vi "WriteItemToExcel.vi"(8 "error in (no error)":errorcluster caption="错误输入（无错误）", 9 "Data":string caption="文本", 10 "保存类型":T1, 11 "report in":refnum<class "NI_report.lvclass"> caption="报表输入") -> (0 "error out":errorcluster caption="错误输出", 3 "report out":refnum<class "NI_report.lvclass"> caption="报表输出")   [LabVIEW 2018]
uses:
  ReportItem.ctl
  <vilib>/Utility/NIReport.llb/NI_report.lvclass
  <vilib>/Utility/NIReport.llb/Append Report Text (str wrap).vi
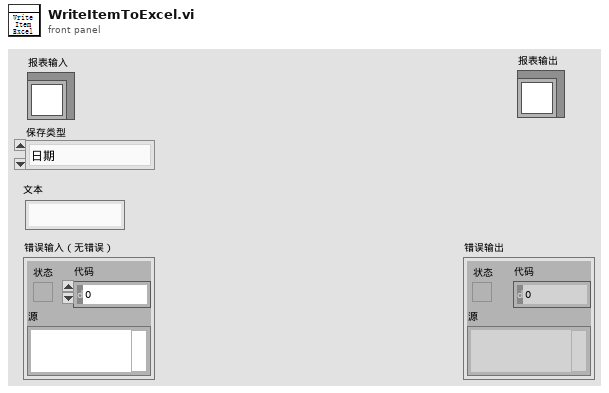
[diagram p1: front panel]
types:
  T1 = typedef "ReportItem.ctl" = enum16{"日期", "激光器编号(Serial)", "功率", "能量", "偏振方向", "偏振度", "脉冲宽度", "脉冲重频", "中心波长", "光谱宽度", "发散角X", "发散角Y", "时间波形路径", "光谱波形路径", "近场图像路径", "远场图像路径", "激光器型号(Type)"}
  T2 = cluster{"position (excel)":cluster{"row":i32, "column":i32}, "name (excel)":string, "bookmark (word)":string}
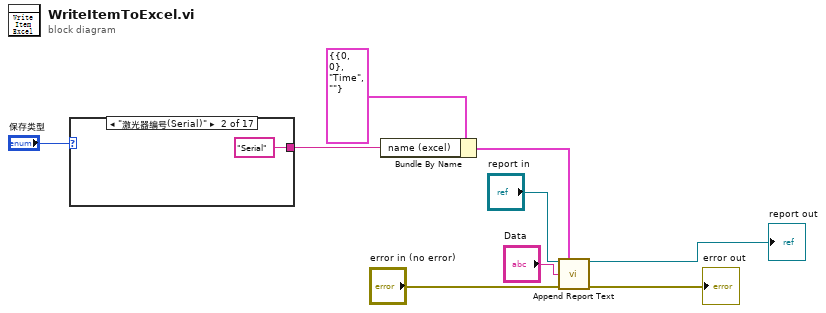
[diagram p0: block diagram]
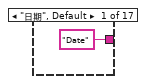
[diagram p2: hidden frame]
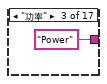
[diagram p3: hidden frame]
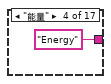
[diagram p4: hidden frame]
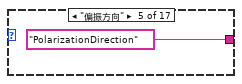
[diagram p5: hidden frame]
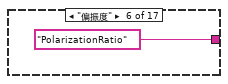
[diagram p6: hidden frame]
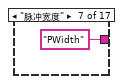
[diagram p7: hidden frame]
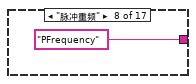
[diagram p8: hidden frame]
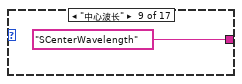
[diagram p9: hidden frame]
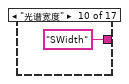
[diagram p10: hidden frame]
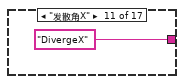
[diagram p11: hidden frame]
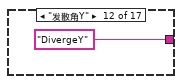
[diagram p12: hidden frame]
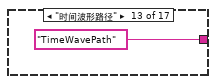
[diagram p13: hidden frame]
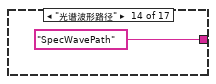
[diagram p14: hidden frame]
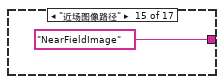
[diagram p15: hidden frame]
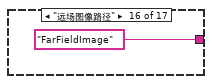
[diagram p16: hidden frame]
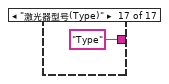
[diagram p17: hidden frame]
diagram:
  n1 = case shown="\"激光器编号(Serial)\"" "保存类型" {
    tunnel: ["Date" "Serial" "Power" "Energy" "PolarizationDirection" "PolarizationRatio" "PWidth" "PFrequency" "SCenterWavelength" "SWidth" "DivergeX" "DivergeY" "TimeWavePath" "SpecWavePath" "NearFieldImage" "FarFieldImage" "Type"] -> w8
    frame "日期", Default {
    }
    frame "激光器编号(Serial)" {
    }
    frame "功率" {
    }
    frame "能量" {
    }
    frame "偏振方向" {
    }
    frame "偏振度" {
    }
    frame "脉冲宽度" {
    }
    frame "脉冲重频" {
    }
    frame "中心波长" {
    }
    frame "光谱宽度" {
    }
    frame "发散角X" {
    }
    frame "发散角Y" {
    }
    frame "时间波形路径" {
    }
    frame "光谱波形路径" {
    }
    frame "近场图像路径" {
    }
    frame "远场图像路径" {
    }
    frame "激光器型号(Type)" {
    }
  }
  n2 = Bundle By Name(cluster=T2 {"position (excel)"={"row"=0, "column"=0}, "name (excel)"="Time", "bookmark (word)"=""} ("MS Office parameters"), "name (excel)"=w8) -> (w7:T2)
  n3 = call-poly <vilib>:"Append Report Text.vi"("report in"="report in", "MS Office parameters"=w7, "text"="Data", "error in (no error)"="error in (no error)") -> ("report out"=→"report out":refnum<class "NI_report.lvclass">, "error out"=→"error out":errorcluster)  [unwired: 8 in, 2 out]
